vi "SSL_accept.vi"(8 "error in (no error)":errorcluster, 11 "SSL in":refnum<class "SSL.lvclass">) -> (0 "error out":errorcluster, 3 "SSL out":refnum<class "SSL.lvclass">)   [LabVIEW 2013, in "SSL_Lib.lvlib" / "SSL.lvclass"]
uses:
  SSL.lvclass
  SSL-Lib/SSL-Lib.lvclass/SSL-Lib.ctl
  SSL.lvclass/SSL.ctl
  SSL-Lib/Read SSL Library Path.vi
  Read Handle.vi
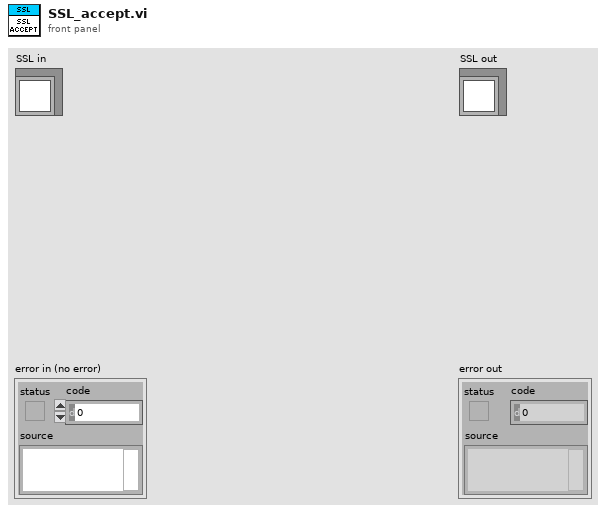
[diagram p1: front panel]
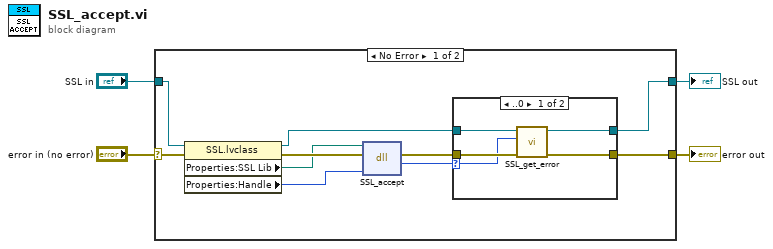
[diagram p0: block diagram]
diagram:
  n1 = case shown="No Error" "error in (no error)" {
    selector: "error in (no error)" -> [w14 w23]
    tunnel: [w7 w23] -> w3
    tunnel: [w5 w22] -> w1
    tunnel: "SSL in" -> [w12 w22]
    frame No Error {
      n2 = property class="SSL.lvclass"(reference=w12, error in=w14) -> (reference out=w6:refnum<class "SSL.lvclass">, error out=w13:errorcluster, "Properties:SSL Lib"=w11:path, "Properties:Handle"=w10:u64)
      n3 = dll-call lib="C:/Program Files (x86)/National Instruments/Shared/nissl/NIssleay32.dll" fn="SSL_accept"(path in=w11, error in=w13, "*SSL"=w10) -> (error out=w8:errorcluster, "return"=w9:i32)  [unwired: 2 in, 1 out]
      n4 = case shown="..0" w9 {
        selector: w9 -> [w15 _]
        tunnel: w8 -> [w19 w21]
        tunnel: [w18 w21] -> w7
        tunnel: w6 -> [w17 w20]
        tunnel: [w16 w20] -> w5
        frame ..0 {
          n5 = call "SSL_get_error.vi"("error in (no error)"=w19, "SSL return code"=w15, "SSL-Lib in"=w17) -> ("error out"=w18:errorcluster, "SSL-Lib out"=w16:refnum<class "SSL.lvclass">)  [unwired: 6 in, 1 out]
        }
        frame Default {
        }
      }
    }
    frame Error {
    }
  }
  "error out" <- w3
  "SSL out" <- w1
